vi "RunOperation.vi"(10 "Inputs":string[](array[string]), 11 "Solution Builder Operation in":refnum<class "sb.lvclass">) -> (1 "Output/Failure":string, 2 "CLI Process Return Code":i32, 3 "Solution Builder Operation out":refnum<class "sb.lvclass">)   [LabVIEW 2019, in "sb.lvclass"]
uses:
  sb.lvclass
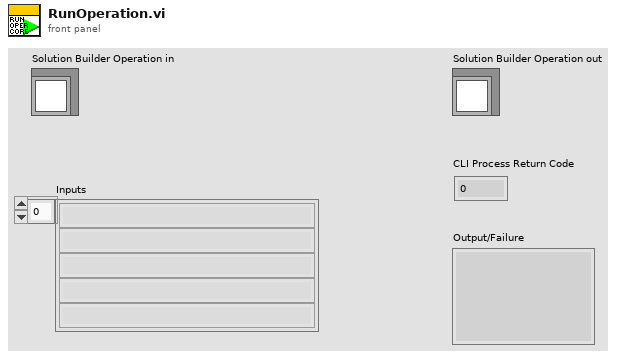
[diagram p1: front panel]
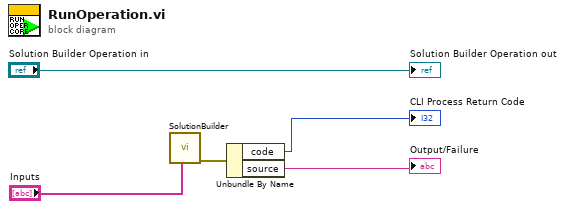
[diagram p0: block diagram]
diagram:
  n1 = call "SolutionBuilder.vi"("Command Line Arguments"="Inputs") -> ("error out"=w3:errorcluster)  [unwired: 8 in, 2 out]
  n2 = Unbundle By Name(w3) -> ("code"=→"CLI Process Return Code":i32, "source"=→"Output/Failure":string)
  "Solution Builder Operation out" <- "Solution Builder Operation in"
